vi "VIMap.vi"(0 "VI Variant":variant, 1 "Value In":variant, 2 "Name":string, 3 "Signal":bool, 4 "VI Name":string) -> (5 "Value Out":variant)   [LabVIEW 2014]
uses:
  Env.global.vi
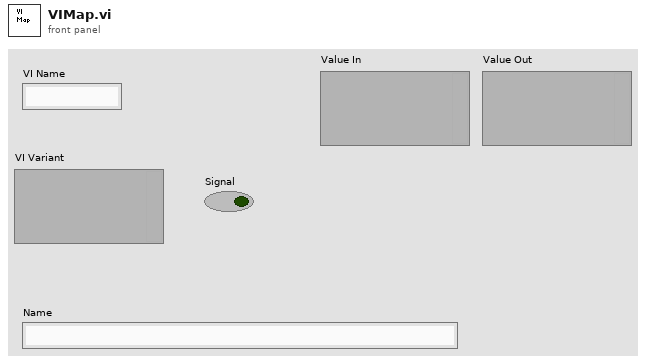
[diagram p1: front panel]
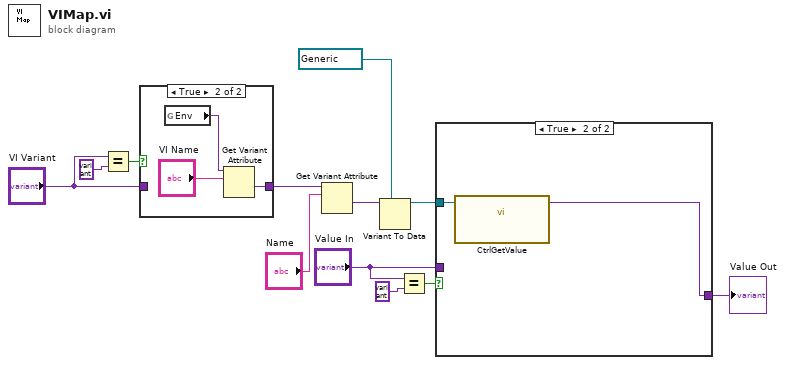
[diagram p0: block diagram]
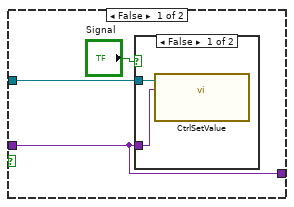
[diagram p3: hidden frame]
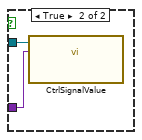
[diagram p4: hidden frame]
diagram:
  n1 = Equal?(x="VI Variant", y=variant ("Env In")) -> (x = y?=w4:bool)
  n2 = case shown="True" w4 {
    tunnel: [w13 w14] -> w2
    tunnel: "VI Variant" -> [w13 _]
    frame False {
    }
    frame True {
      n3 = global read "Env.global.vi" "Env"() -> (w15:variant)
      n4 = Get Variant Attribute(Variant=w15, name="VI Name") -> (value=w14:variant)  [unwired: 2 in, 3 out]
    }
  }
  n5 = Get Variant Attribute(Variant=w2, name="Name") -> (value=w11:variant)  [unwired: 2 in, 3 out]
  n6 = Variant To Data(type=refnum<vi> refnum ("reference"), Variant=w11) -> (data=w8:refnum<vi>)  [unwired: 1 in, 1 out]
  n7 = Equal?(x="Value In", y=variant ("Value In")) -> (x = y?=w1:bool)
  n8 = case shown="True" w1 {
    tunnel: w8 -> [w19 w25]
    tunnel: [w18 w24] -> w7
    tunnel: "Value In" -> [w18 _]
    frame False {
      n9 = case shown="False" "Signal" {
        tunnel: w19 -> [w21 w23]
        tunnel: w18 -> [w20 w22]
        frame False {
          n10 = call "CtrlSetValue.vi"("variant"=w20, "reference"=w21) -> ()  [unwired: 2 in, 1 out]
        }
        frame True {
          n11 = call "CtrlSignalValue.vi"("variant"=w22, "reference"=w23) -> ()  [unwired: 2 in, 1 out]
        }
      }
    }
    frame True {
      n12 = call "CtrlGetValue.vi"("reference"=w25) -> ("variant"=w24:variant)  [unwired: 1 in, 3 out]
    }
  }
  "Value Out" <- w7
